vi "esp301 set move to hard limit.vi"(7 "Seperator in":string, 8 "error in (no error)":errorcluster, 9 "Args":string[](array[string]), 10 "String":string, 11 "ESP301 in":refnum<class "ESP301.lvclass">) -> (0 "error out":errorcluster, 2 "new commands":string, 3 "ESP301 out":refnum<class "ESP301.lvclass">)   [LabVIEW 2020, in "ESP301.lvclass"]
uses:
  ESP301.lvclass
  Hardware limit.ctl
  shared/OnOffTypeDef.ctl
  ESP301.lvclass/ESP301.ctl
  shared/CompressAndUpdate(Poly)/CompressAndUpdate(Enum).vi
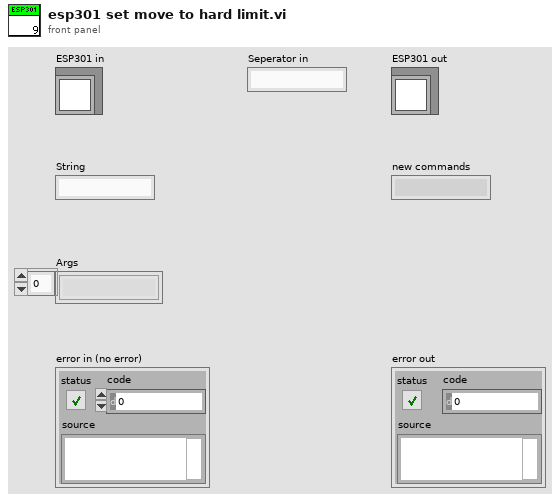
[diagram p1: front panel]
types:
  T1 = typedef "OnOffTypeDef.ctl" = enum16{"off", "on"}
  T2 = typedef "Hardware limit.ctl" = enum16{"pos", "neg"}
  T3 = enum16{"Not referenced", "Homing", "Moving", "Ready"}
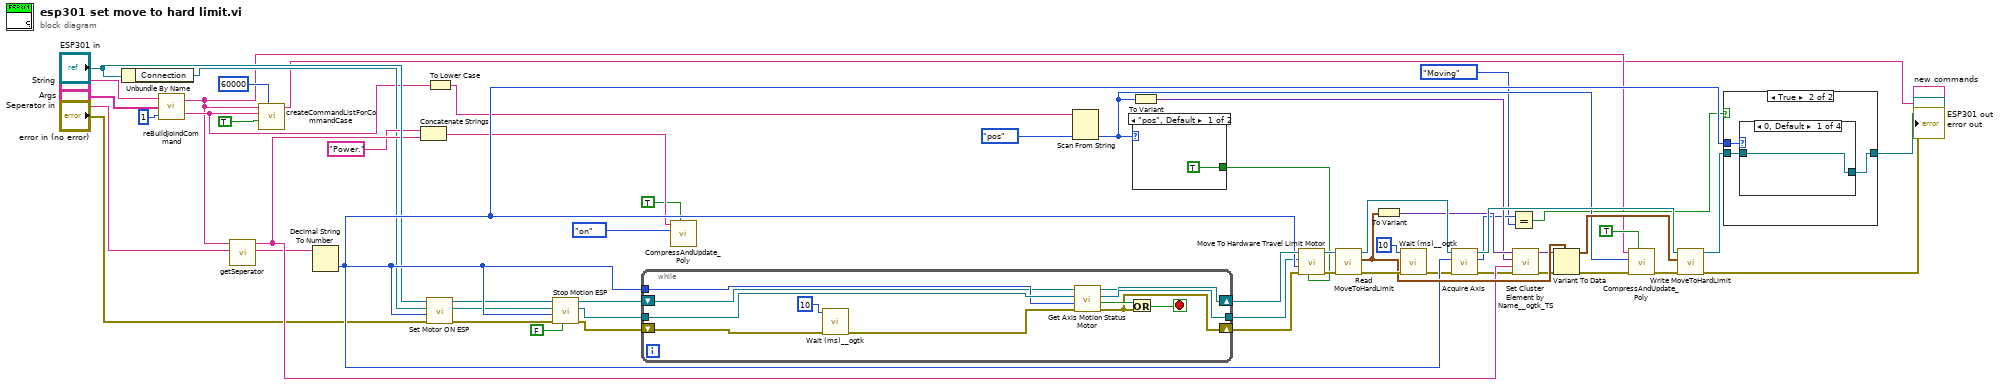
[diagram p0: block diagram]
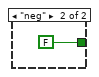
[diagram p2: hidden frame]
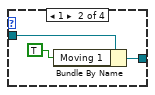
[diagram p4: hidden frame]
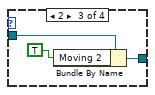
[diagram p5: hidden frame]
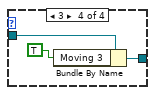
[diagram p6: hidden frame]
diagram:
  n1 = Unbundle By Name("ESP301 in") -> ("Connection"=w26:refnum<visa-resource-name>)
  n2 = call "reBuildJoindCommand.vi"("number of group elements (0)"=1, "Args"="Args", "Command 2"="String") -> ("Arg"=w9:string, "Command"=w8:string)
  n3 = call "getSeperator.vi"("Channel Seperator (\"\")"="Seperator in", "Command"=w8) -> ("Channel"=w6:string, "Seperator (e.g. \"Channel1\")"=w34:string)  [unwired: 8 in]
  n4 = call "createCommandListForCommandCase.vi"("timeout (optional)"=60000, "immediate Check (only once)"=TRUE, "setvalue"=w9, "command"=w8) -> ("new commands"=→"new commands":string)  [unwired: 7 in]
  n5 = Decimal String To Number(string=w6) -> (number=w43:i32)  [unwired: 2 in, 1 out]
  n6 = Concatenate Strings("Power." ("string"), w34) -> (w32:string)
  n7 = call-dynamic "Set Motor ON ESP.vi"("error in (no error)"="error in (no error)", "Axis (1)"=w43, "VISA resource name"=w26, "ESP301 in"="ESP301 in") -> ("error out"=w29:errorcluster, "VISA resource name out"=w27:refnum<visa-resource-name>, "ESP301 out"=w39:refnum<class "ESP301.lvclass">)  [unwired: 5 in]
  n8 = To Lower Case(string=w9) -> (all lower case string=w24:string)
  n9 = call-dynamic "Stop Motion ESP.vi"("Stop all axes (F)"=FALSE, "error in (no error)"=w29, "Axis (1)"=w43, "VISA resource name"=w27, "ESP301 in"=w39) -> ("error out"=w14:errorcluster, "VISA resource name out"=w15:refnum<visa-resource-name>, "ESP301 out"=w40:refnum<class "ESP301.lvclass">)  [unwired: 4 in]
  n10 = while {
    tunnel: w15 -> [w67]
    tunnel: w43 -> [w66]
    tunnel: [w64] -> w42
    shift-right: [w62] -> w41
    shift-left: w14 -> [w65]
    shift-right: [w59] -> w45
    shift-left: w40 -> [w60]
    stop <- w61 stop-if-true
    n11 = call <userlib>:"Wait (ms)__ogtk.vi"("error in (no error)"=w65, "milliseconds to wait"=u32 10) -> ("error out"=w58:errorcluster)  [unwired: 8 in, 1 out]
    n12 = call-dynamic "Get Axis Motion Status Motor.vi"("error in (no error)"=w58, "Axis (1)"=w66, "VISA resource name"=w67, "ESP301 in"=w60) -> ("error out"=w62:errorcluster, "Motion Done"=w63:bool, "VISA resource name out"=w64:refnum<visa-resource-name>, "ESP301 out"=w59:refnum<class "ESP301.lvclass">)  [unwired: 4 in]
    n13 = Or(x=w63, y=w62) -> (x .or. y?=w61:bool)
  }
  n14 = call-poly "CompressAndUpdate_Poly.vi"("force CVT update (false)"=TRUE ("force CVT update"), "enum variant"=OnOffTypeDef."on" ("Axis 1"), "command or variable name"=w32) -> ()  [unwired: 8 in, 1 out]
  n15 = Scan From String(input string=w24, default 1=Hardware_limit."pos" ("Axis 1")) -> (output 1=w25:T2)  [unwired: 3 in, 3 out]
  n16 = case shown="\"pos\", Default" w25 {
    tunnel: [TRUE ("immediate Check (only once)") FALSE ("immediate Check (only once)")] -> w44
    frame "pos", Default {
    }
    frame "neg" {
    }
  }
  n17 = To Variant(anything=w25) -> (Variant=w36:variant)
  n18 = call-dynamic "Move To Hardware Travel Limit Motor.vi"("Move Direction (+)"=w44, "error in (no error)"=w41, "Axis (1)"=w43, "VISA resource name"=w42, "ESP301 in"=w45) -> ("error out"=w48:errorcluster, "ESP301 out"=w46:refnum<class "ESP301.lvclass">)  [unwired: 4 in, 1 out]
  n19 = call "Read MoveToHardLimit.vi"("error in (no error)"=w48, "ESP301 in"=w46) -> ("error out"=w54:errorcluster, "MoveToHardLimit"=w53:cluster{"Axis 1":T2, "Axis 2":T2, "Axis 3":T2}, "ESP301 out"=w55:refnum<class "ESP301.lvclass">)  [unwired: 7 in]
  n20 = To Variant(anything=w53) -> (Variant=w37:variant)
  n21 = call <userlib>:"Wait (ms)__ogtk.vi"("error in (no error)"=w54, "milliseconds to wait"=u32 10) -> ("error out"=w22:errorcluster)  [unwired: 8 in, 1 out]
  n22 = call "Acquire Axis.vi"("error in (no error)"=w22, "Axis"=w43, "Object in"=w55) -> ("error out"=w12:errorcluster, "Status"=w20:T3, "Object out"=w56:refnum<class "ESP301.lvclass">)  [unwired: 4 in, 2 out]
  n23 = Equal?(x=w20, y=T3."Moving" ("Axis 3")) -> (x = y?=w21:bool)
  n24 = call "Set Cluster Element by Name__ogtk_TS.vi"("error in (no error)"=w12, "Element Name (\"\": New Element Data Name)"=w34, "New Element Value"=w36, "Cluster"=w37) -> ("error out"=w16:errorcluster, "VCluster out"=w17:variant)  [unwired: 5 in, 1 out]
  n25 = Variant To Data(error in=w16, type=w53, Variant=w17) -> (data=w49:cluster{"Axis 1":T2, "Axis 2":T2, "Axis 3":T2}, error out=w18:errorcluster)
  n26 = call-poly "CompressAndUpdate_Poly.vi"("force CVT update (false)"=TRUE ("force CVT update"), "error in"=w18, "enum variant"=w25, "command or variable name"=w8) -> ("error out"=w51:errorcluster)  [unwired: 7 in]
  n27 = call "Write MoveToHardLimit.vi"("error in (no error)"=w51, "MoveToHardLimit"=w49, "ESP301 in"=w56) -> ("error out"=→"error out":errorcluster, "ESP301 out"=w50:refnum<class "ESP301.lvclass">)  [unwired: 7 in]
  n28 = case shown="True" w21 {
    tunnel: w43 -> [_ w73]
    tunnel: w50 -> [w70 w72]
    tunnel: [w70 w71] -> w7
    frame False {
    }
    frame True {
      n29 = case shown="0, Default" w73 {
        tunnel: w72 -> [w74 w77 w80 w83]
        tunnel: [w74 w76 w79 w82] -> w71
        frame 0, Default {
        }
        frame 1 {
          n30 = Bundle By Name(cluster=w77, "Moving 1"=TRUE) -> (w76:refnum<class "ESP301.lvclass">)
        }
        frame 2 {
          n31 = Bundle By Name(cluster=w80, "Moving 2"=TRUE) -> (w79:refnum<class "ESP301.lvclass">)
        }
        frame 3 {
          n32 = Bundle By Name(cluster=w83, "Moving 3"=TRUE) -> (w82:refnum<class "ESP301.lvclass">)
        }
      }
    }
  }
  "ESP301 out" <- w7
